vi "get_all_output_names.vi"(8 "error in (no error)":errorcluster, 11 "VISA resource name":refnum<visa-resource-name>) -> (0 "error out":errorcluster, 2 "All ouput names":string[](array[string]), 3 "VISA resource name out":refnum<visa-resource-name>)   [LabVIEW 2018, in "Inficon IC6.lvlib"]
doc: "Update all output names."
uses:
  <instrlib>/Inficon IC6/Inficon IC6.lvlib
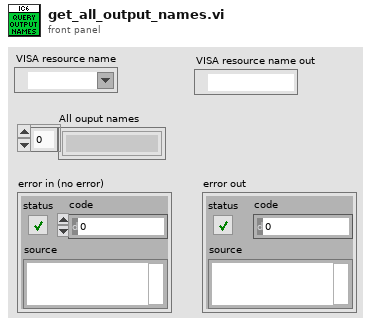
[diagram p1: front panel]
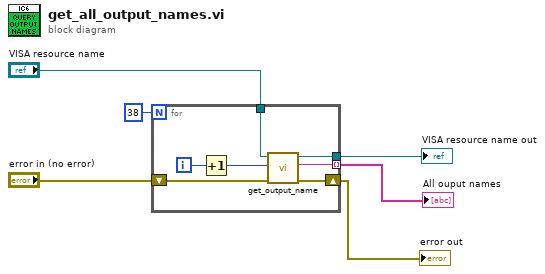
[diagram p0: block diagram]
diagram:
  n1 = for {
    N: 38 -> [_]
    tunnel: "VISA resource name" -> [w11]
    tunnel: [w10] -> w3
    shift-right: [w8] -> w6
    shift-left: "error in (no error)" -> [w9]
    tunnel: [w7] -> w1 mode=indexing
    i -> [w13]
    n2 = Increment(x=w13) -> (x+1=w12:i32)
    n3 = call <instrlib>:"get_output_name.vi"("error in (no error)"=w9, "output number"=w12, "VISA resource name"=w11) -> ("error out"=w8:errorcluster, "output name"=w7:string, "VISA resource name out"=w10:refnum<visa-resource-name>)  [unwired: 6 in]
  }
  "error out" <- w6
  "All ouput names" <- w1
  "VISA resource name out" <- w3
